vi "ErrorHandling.Initialization.vi"(8 "error in":errorcluster, 10 "ErrorBasePath":path=path "D:/Data/BioReactor/ErrorLog", 11 "ErrorHandling(optional)":refnum<data-value>) -> (0 "error out":errorcluster, 3 "ErrorHandling out":refnum<data-value>)   [LabVIEW 2016, in "ErrorHandling.lvclass"]
doc: "Initializes the ErrorHandling Object and loads custom error codes, saves them to the ErrorHandling.lvclass and loads occured errors from the errorlog file. (Saves ErrorHandler Ref to the ObjRefTable)\n\n23.08.2016, Andreas Elmiger"
uses:
  ErrorHandling.lvclass
  ErrorHandling.lvclass/ErrorHandling.ctl
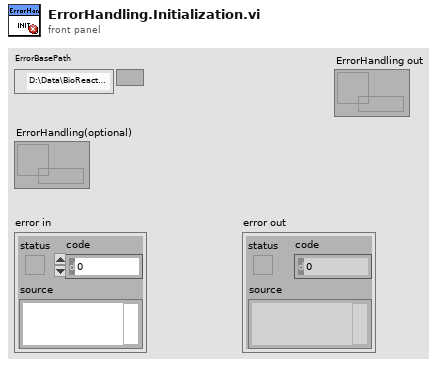
[diagram p1: front panel]
types:
  T1 = enum16{"open", "replace", "create", "open or create", "replace or create", "replace or create with confirmation"}
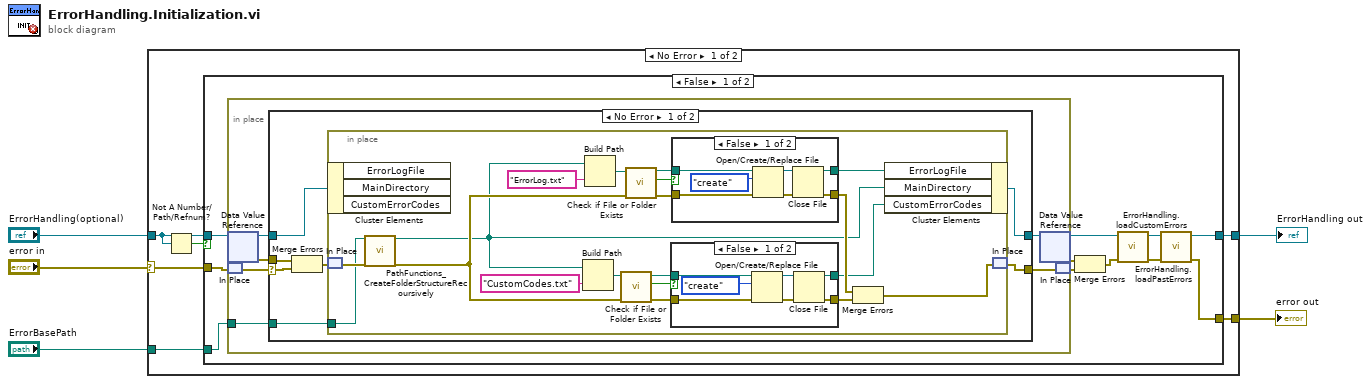
[diagram p0: block diagram]
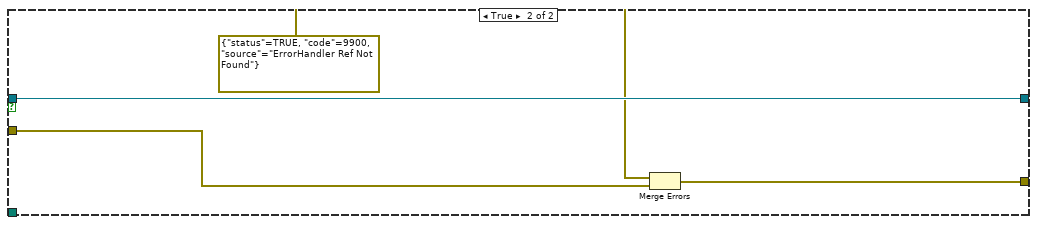
[diagram p5: hidden frame]
diagram:
  n1 = case shown="No Error" "error in" {
    selector: "error in" -> [w6 w80]
    tunnel: [w11 w80] -> w4
    tunnel: [w10 w79] -> w3
    tunnel: "ErrorHandling(optional)" -> [w7 w79]
    tunnel: "ErrorBasePath" -> [w9 _]
    frame No Error {
      n2 = Not A Number/Path/Refnum?(number/path/refnum=w7) -> (NaN/Path/Refnum?=w8:bool)
      n3 = case shown="False" w8 {
        tunnel: [w16 w76] -> w11
        tunnel: w7 -> [w22 w78]
        tunnel: w6 -> [w21 w75]
        tunnel: [w17 w78] -> w10
        tunnel: w9 -> [w18 _]
        frame False {
          n4 = in-place {
            in-place-border: w18 -> [w24]
            n5 = in-place-dvr #1(w22) -> (w28:refnum<class "ErrorHandling.lvclass">, w26:errorcluster)
            n6 = in-place-match #2(w21) -> (w27:errorcluster)
            n7 = case shown="No Error" w27 {
              selector: w27 -> [w33 w73]
              tunnel: [w34 w74] -> w23
              tunnel: w28 -> [w35 w74]
              tunnel: w26 -> [w32 _]
              tunnel: [w30 w73] -> w25
              tunnel: w24 -> [w29 _]
              frame No Error {
                n8 = Merge Errors(w32, w33) -> (w31:errorcluster)
                n9 = in-place {
                  in-place-border: w29 -> [w53]
                  n10 = in-place-cluster #3(w35) -> ()  [unwired: 3 out]
                  n11 = in-place-match #4(w31) -> (w54:errorcluster)
                  n12 = call "PathFunctions_CreateFolderStructureRecoursively.vi"("Path"=w53, "ErrorIn"=w54) -> ("Path(dup)"=w39:path, "ErrorOut"=w45:errorcluster)  [unwired: 15 in, 1 out]
                  n13 = Build Path(base path=w39, name or relative path="CustomCodes.txt") -> (appended path=w41:path)
                  n14 = Build Path(base path=w39, name or relative path="ErrorLog.txt") -> (appended path=w38:path)
                  n15 = call <vilib>:"Check if File or Folder Exists.vi"("error in (no error)"=w45, "path"=w41) -> ("error out"=w47:errorcluster, "file or folder exists?"=w46:bool, "dup path"=w48:path)  [unwired: 7 in]
                  n16 = call <vilib>:"Check if File or Folder Exists.vi"("error in (no error)"=w45, "path"=w38) -> ("error out"=w43:errorcluster, "file or folder exists?"=w37:bool, "dup path"=w44:path)  [unwired: 7 in]
                  n17 = case shown="False" w46 {
                    tunnel: w47 -> [w61 w63]
                    tunnel: w48 -> [w55 w62]
                    tunnel: [w57 w63] -> w50
                    tunnel: [w56 w62] -> w49
                    frame False {
                      n18 = Open/Create/Replace File(file path (use dialog)=w55, error in=w61, operation (0:open)=T1."create") -> (refnum out=w58:refnum<file>, error out=w59:errorcluster)  [unwired: 3 in, 1 out]
                      n19 = Close File(refnum=w58, error in=w59) -> (path=w56:path, error out=w57:errorcluster)
                    }
                    frame True {
                    }
                  }
                  n20 = case shown="False" w37 {
                    tunnel: w43 -> [w70 w72]
                    tunnel: w44 -> [w64 w71]
                    tunnel: [w66 w72] -> w51
                    tunnel: [w65 w71] -> w36
                    frame False {
                      n21 = Open/Create/Replace File(file path (use dialog)=w64, error in=w70, operation (0:open)=T1."create") -> (refnum out=w67:refnum<file>, error out=w68:errorcluster)  [unwired: 3 in, 1 out]
                      n22 = Close File(refnum=w67, error in=w68) -> (path=w65:path, error out=w66:errorcluster)
                    }
                    frame True {
                    }
                  }
                  n23 = Merge Errors(w51, w50) -> (w52:errorcluster)
                  n24 = in-place-cluster #3("ErrorLogFile"=w36, "MainDirectory"=w39, "CustomErrorCodes"=w49) -> (w34:refnum<class "ErrorHandling.lvclass">)
                  n25 = in-place-match #4(w52) -> (w30:errorcluster)
                }
              }
              frame Error {
              }
            }
            n26 = in-place-dvr #1(w23) -> (w12:refnum<data-value>, w19:errorcluster)
            n27 = in-place-match #2(w25) -> (w20:errorcluster)
          }
          n28 = Merge Errors(w19, w20) -> (w15:errorcluster)
          n29 = call "ErrorHandling.loadCustomErrors.vi"("error in (no error)"=w15, "ErrorHandling in"=w12) -> ("error out"=w14:errorcluster, "ErrorHandling out"=w13:refnum<data-value>)  [unwired: 8 in]
          n30 = call "ErrorHandling.loadPastErrors.vi"("error in (no error)"=w14, "ErrorHandling in"=w13) -> ("error out"=w16:errorcluster, "ErrorHandling out"=w17:refnum<data-value>)  [unwired: 8 in]
        }
        frame True {
          n31 = Merge Errors(errorcluster {"status"=TRUE, "code"=9900, "source"="ErrorHandler Ref Not Found"} ("error IO"), w75) -> (w76:errorcluster)
        }
      }
    }
    frame Error {
    }
  }
  "ErrorHandling out" <- w3
  "error out" <- w4
